vi "Optical_Image.vi"() -> ()   [LabVIEW 2022 SP3]
panel:
  out "Image Size (cm)":dbl
  in  "Object Size (cm)":dbl
  out "Magnification":dbl
  out "Image distance (cm)":dbl
  in  "Focal length (cm)":dbl
  in  "Object location (cm)":dbl
  # "Optical_Image:\nFor an object placed in front of a curved mirror,\nenter the distance of the object from the mirror,\nthe focal length of the mirror, and the size of the \nobject."
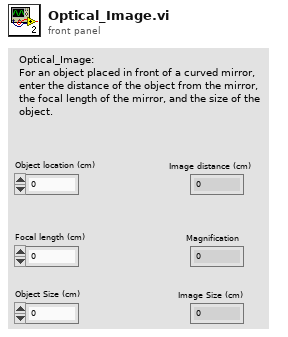
[diagram p1: front panel]
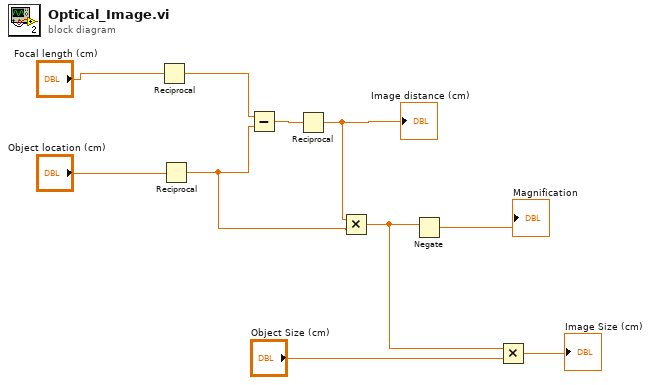
[diagram p0: block diagram]
diagram:
  n1 = Reciprocal(x="Focal length (cm)") -> (1/x=w8:dbl)
  n2 = Reciprocal(x="Object location (cm)") -> (1/x=w5:dbl)
  n3 = Subtract(x=w8, y=w5) -> (x-y=w7:dbl)
  n4 = Reciprocal(x=w7) -> (1/x=w6:dbl)
  "Image distance (cm)" <- w6
  n5 = Multiply(x=w6, y=w5) -> (x*y=w2:dbl)
  n6 = Negate(x=w2) -> (-x=→"Magnification":dbl)
  n7 = Multiply(x=w2, y="Object Size (cm)") -> (x*y=→"Image Size (cm)":dbl)
